vi "VI Server_ABORT_if_ClusterEmpty.vi"(4 "VI Server.RefsCluster":T1, 5 "Calling VI Path":path) -> (1 "VI Server.RefsCluster.DUP":T1)   [LabVIEW 2020]
uses:
  VI Server_TypeDefs/VI Server_RefsCluster.ctl
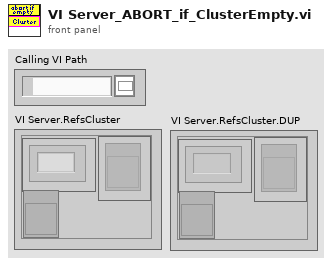
[diagram p1: front panel]
types:
  T1 = typedef "VI Server_RefsCluster.ctl" = cluster{"Labels":string[], "Refs":refnum<vi>[], "VI Ref":refnum<vi>}
  T2 = enum32{"Invalid", "Standard", "Closed", "Hidden", "Minimized", "Maximized"}
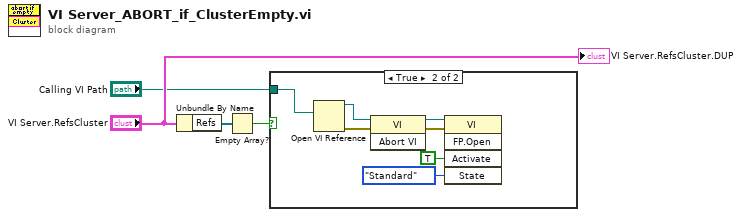
[diagram p0: block diagram]
diagram:
  n1 = Unbundle By Name("VI Server.RefsCluster") -> ("Refs"=w4:refnum<vi>[])
  n2 = Empty Array?(array=w4) -> (empty?=w3:bool)
  n3 = case shown="True" w3 {
    tunnel: "Calling VI Path" -> [_ w5]
    frame False {
    }
    frame True {
      n4 = Open VI Reference(vi path=w5) -> (vi reference=w10:refnum<vi>, error out=w11:errorcluster)  [unwired: 5 in]
      n5 = invoke class="VI" method="Abort VI"(reference=w10, error in=w11) -> (reference out=w8:refnum<vi>, error out=w9:errorcluster)  [unwired: 1 in, 1 out]
      n6 = invoke class="VI" method="FP.Open"(reference=w8, error in=w9, "Activate"=TRUE ("Activate?"), "State"=T2."Standard") -> ()  [unwired: 1 in, 5 out]
    }
  }
  "VI Server.RefsCluster.DUP" <- "VI Server.RefsCluster"
